vi "Deserialize Data.vi"(8 "error in (no error)":errorcluster, 11 "Flat Data in":string) -> (0 "error out":errorcluster, 3 "Process Data out":T1)   [LabVIEW 2020, in "Optitrack.lvlib"]
doc: "Version 0.1"
uses:
  <vilib>/ADAS Record/CustomDataTypes/Optitrack/Optitrack.lvlib
  5e2451cd-7b8c-4079-9add-41a600a01e16.vi
  <vilib>/ADAS Record/CustomDataTypes/Optitrack/Process Data.ctl
  <vilib>/ADAS Record/IODataPEF/CfgMgr/FlatFormat.ctl
  Projects/NI AzDO/Mercedes-MPIC-201077/Record_MPIC3/mercedes-record-mpic3-201077/software-record-plugins/labview-2020/src/shared/TypeDef-Optitrack-RigidBody.ctl
  Projects/NI AzDO/Mercedes-MPIC-201077/Record_MPIC3/mercedes-record-mpic3-201077/software-record-plugins/labview-2020/src/shared/TypeDef-Optitrack-MarkerPoint.ctl
  Projects/NI AzDO/Mercedes-MPIC-201077/Record_MPIC3/mercedes-record-mpic3-201077/software-record-plugins/labview-2020/src/shared/TypeDef-Optitrack-MarkerSet.ctl
  Projects/NI AzDO/Mercedes-MPIC-201077/Record_MPIC3/mercedes-record-mpic3-201077/software-record-plugins/labview-2020/src/shared/TypeDef-Optitrack-LabeledMarker.ctl
  Projects/NI AzDO/Mercedes-MPIC-201077/Record_MPIC3/mercedes-record-mpic3-201077/software-record-plugins/labview-2020/src/shared/TypeDef-Optitrack-TrackedData.ctl
  Projects/NI AzDO/Mercedes-MPIC-201077/Record_MPIC3/mercedes-record-mpic3-201077/software-record-plugins/labview-2020/src/shared/TypeDef-Optitrack-FrameData.ctl
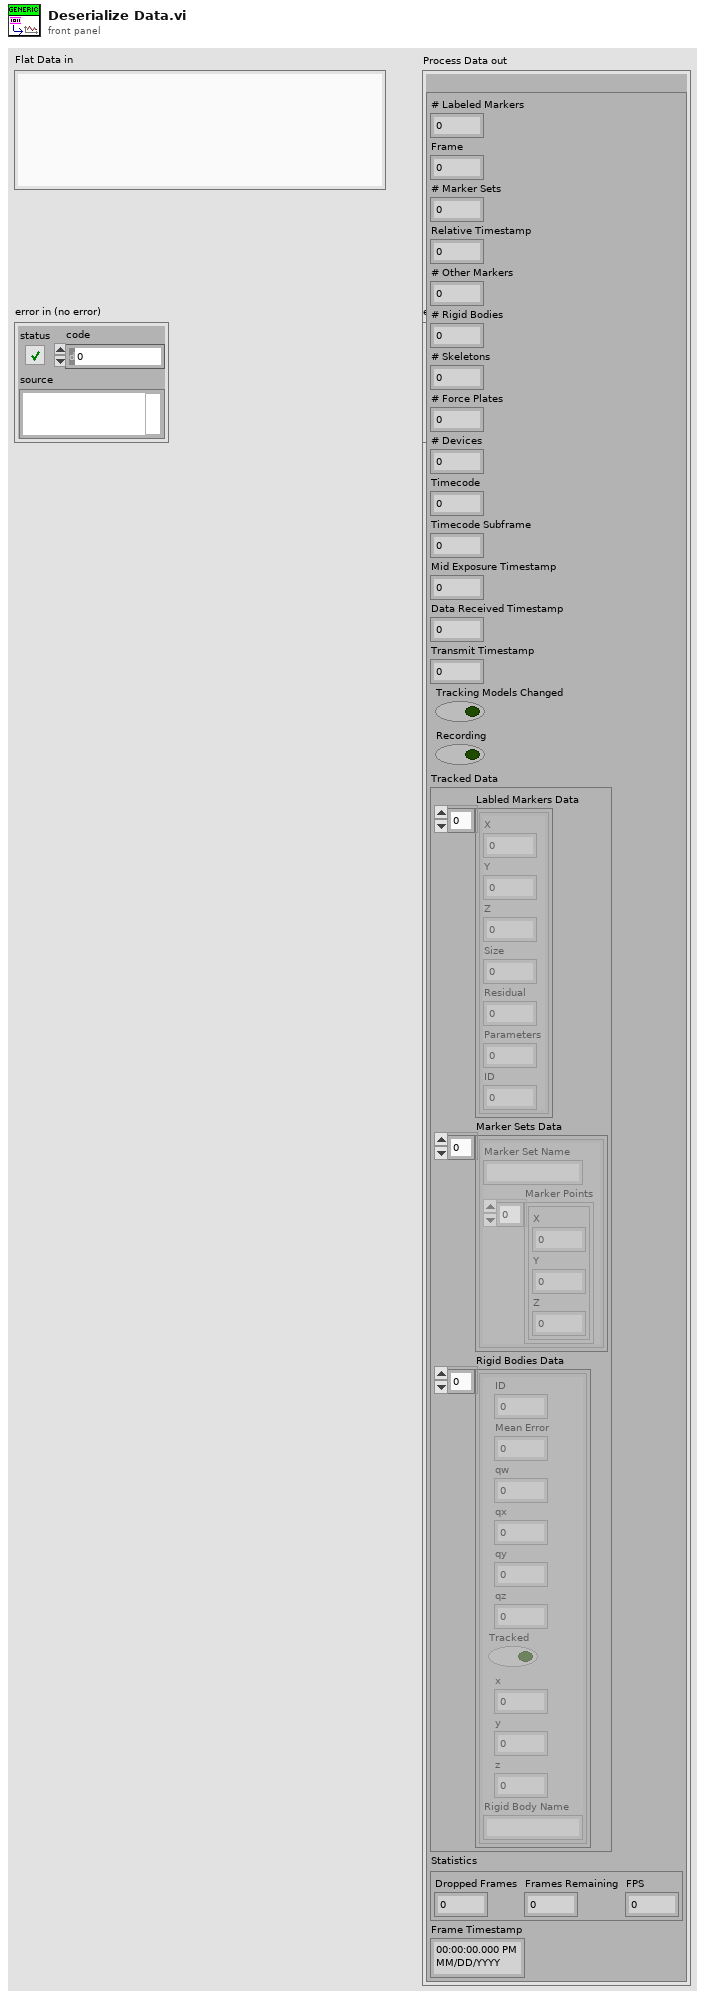
[diagram p1: front panel]
types:
  T1 = typedef "Optitrack.lvlib/Process Data.ctl" = cluster{"OptitrackFrame":T2}
  T2 = typedef "TypeDef-Optitrack-FrameData.ctl" = cluster{"# Labeled Markers":i32, "Frame":i32, "# Marker Sets":i32, "Relative Timestamp":dbl, "# Other Markers":i32, "# Rigid Bodies":i32, "# Skeletons":i32, "# Force Plates":i32, "# Devices":i32, "Timecode":u32, "Timecode Subframe":u32, "Mid Exposure Timestamp":u64, "Data Received Timestamp":u64, "Transmit Timestamp":u64, "Tracking Models Changed":bool, "Recording":bool, "Tracked Data":T3, "Statistics":cluster{"Dropped Frames":i32, "Frames Remaining":i32, "FPS":dbl}, "Frame Timestamp":timestamp}
  T3 = typedef "TypeDef-Optitrack-TrackedData.ctl" = cluster{"Labled Markers Data":T4[], "Marker Sets Data":T5[], "Rigid Bodies Data":T7[]}
  T4 = typedef "TypeDef-Optitrack-LabeledMarker.ctl" = cluster{"X":sgl, "Y":sgl, "Z":sgl, "Size":sgl, "Residual":sgl, "Parameters":i16, "ID":i32}
  T5 = typedef "TypeDef-Optitrack-MarkerSet.ctl" = cluster{"Marker Set Name":string, "Marker Points":T6[]}
  T6 = typedef "TypeDef-Optitrack-MarkerPoint.ctl" = cluster{"X":sgl, "Y":sgl, "Z":sgl}
  T7 = typedef "TypeDef-Optitrack-RigidBody.ctl" = cluster{"ID":i32, "Mean Error":sgl, "qw":sgl, "qx":sgl, "qy":sgl, "qz":sgl, "Tracked":bool, "x":sgl, "y":sgl, "z":sgl, "Rigid Body Name":string}
  T8 = typedef "FlatFormat.ctl" = enum32{"Auto", "PEF", "GFB (Apache)", "GFB", "JSON", "Readable JSON", "LV String", "Reserved", "LV Native"}
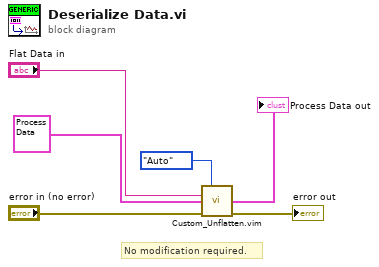
[diagram p0: block diagram]
diagram:
  # "No modification required."
  n1 = call "Custom_Unflatten.vim"("Flat Format"=FlatFormat."Auto", "Flat Data"="Flat Data in", "Data (type/default value)"=T1 {"OptitrackFrame"={"# Labeled Markers"=0, "Frame"=0, "# Marker Sets"=0, "Relative Timestamp"=0.0, "# Other Markers"=0, "# Rigid Bodies"=0, "# Skeletons"=0, "# Force Plates"=0, "# Devices"=0, "Timecode"=0, "Timecode Subframe"=0, "Mid Exposure Timestamp"=0, "Data Received Timestamp"=0, "Transmit Timestamp"=0, "Tracking Models Changed"=FALSE, "Recording"=FALSE, "Tracked Data"={"Labled Markers Data"=[], "Marker Sets Data"=[], "Rigid Bodies Data"=[]}, "Statistics"={"Dropped Frames"=0, "Frames Remaining"=0, "FPS"=0.0}, "Frame Timestamp"=timestamp(0 s since 1904-01-01)}} ("Byte Array in"), "error in (no error)"="error in (no error)") -> ("Data"=→"Process Data out":T1, "Error (out)"=→"error out":errorcluster)  [unwired: 10 in]
